vi "choose_data_for_spectrum_graph.vi"(1 "Data Type":T3(ring), 2 "Data cluster":T2) -> (0 "Data for SpectrumGraph":T1(array[cluster]))   [LabVIEW 2017]
uses:
  controls/Data.ctl
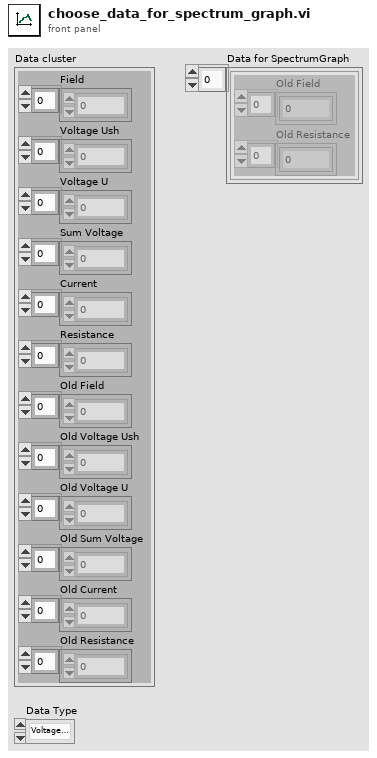
[diagram p1: front panel]
types:
  T1 = cluster{"Old Field":dbl[], "Old Resistance":dbl[]}[]
  T2 = typedef "Data.ctl" = cluster{"Field":dbl[], "Voltage Ush":dbl[], "Voltage U":dbl[], "Sum Voltage":dbl[], "Current":dbl[], "Resistance":dbl[], "Old Field":dbl[], "Old Voltage Ush":dbl[], "Old Voltage U":dbl[], "Old Sum Voltage":dbl[], "Old Current":dbl[], "Old Resistance":dbl[]}
  T3 = enum16{"Voltage Ush, V", "Voltage U, V", "Sum Voltage, V", "Current, mA", "Resistance, Ohm"}
  T4 = cluster{"Old Field":dbl[], "Old Resistance":dbl[]}
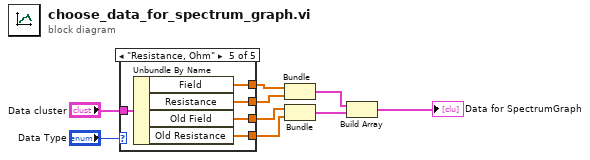
[diagram p0: block diagram]
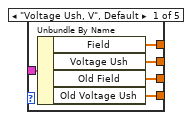
[diagram p2: hidden frame]
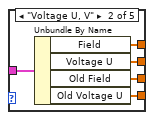
[diagram p3: hidden frame]
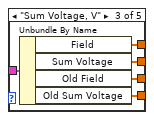
[diagram p4: hidden frame]
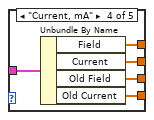
[diagram p5: hidden frame]
diagram:
  n1 = case shown="\"Resistance, Ohm\"" "Data Type" {
    tunnel: "Data cluster" -> [w14 w19 w24 w29 w32]
    tunnel: [w13 w18 w23 w28 w34] -> w6
    tunnel: [w12 w17 w22 w27 w33] -> w7
    tunnel: [w11 w16 w21 w26 w31] -> w8
    tunnel: [w10 w15 w20 w25 w30] -> w9
    frame "Voltage Ush, V", Default {
      n2 = Unbundle By Name(w14) -> ("Field"=w13:dbl[], "Voltage Ush"=w12:dbl[], "Old Field"=w11:dbl[], "Old Voltage Ush"=w10:dbl[])
    }
    frame "Voltage U, V" {
      n3 = Unbundle By Name(w19) -> ("Field"=w18:dbl[], "Voltage U"=w17:dbl[], "Old Field"=w16:dbl[], "Old Voltage U"=w15:dbl[])
    }
    frame "Sum Voltage, V" {
      n4 = Unbundle By Name(w24) -> ("Field"=w23:dbl[], "Sum Voltage"=w22:dbl[], "Old Field"=w21:dbl[], "Old Sum Voltage"=w20:dbl[])
    }
    frame "Current, mA" {
      n5 = Unbundle By Name(w29) -> ("Field"=w28:dbl[], "Current"=w27:dbl[], "Old Field"=w26:dbl[], "Old Current"=w25:dbl[])
    }
    frame "Resistance, Ohm" {
      n6 = Unbundle By Name(w32) -> ("Field"=w34:dbl[], "Resistance"=w33:dbl[], "Old Field"=w31:dbl[], "Old Resistance"=w30:dbl[])
    }
  }
  n7 = Bundle("Field"=w6, "Resistance"=w7) -> (w1:cluster{"Field":dbl[], "Resistance":dbl[]})  [unwired: 1 in]
  n8 = Bundle("Old Field"=w8, "Old Resistance"=w9) -> (w2:T4)  [unwired: 1 in]
  n9 = Build Array(w1, w2) -> (→"Data for SpectrumGraph":T1)
